vi "GF_Fire_VFandUF.vi"(0 "VF task":refnum<k21>, 1 "Fake Form index":i32, 2 "Preflash Index":i32, 3 "Preflash Width\\Lead":i32=2000, 5 "VF trig array size":i32, 7 "UF task":refnum<k21>, 9 "UF trig array size":i32, 11 "error in":errorcluster, 12 "Spectro Trig Index":i32, 13 "VF Trig Channel":refnum<k21>="USB_TurnOffBProbeRelay_P0_4") -> (15 "error out":errorcluster)   [LabVIEW 2009]
panel:
  out "Very Fast  Fire Waveform":digitalwaveform[](graph)
  out "Ultra Fast  Fire Waveform":digitalwaveform[](graph)
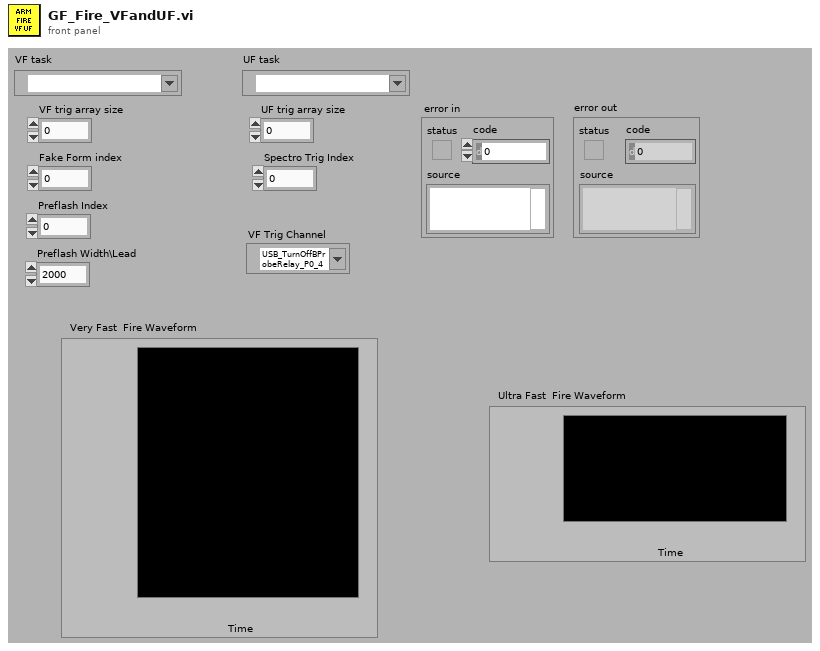
[diagram p1: front panel]
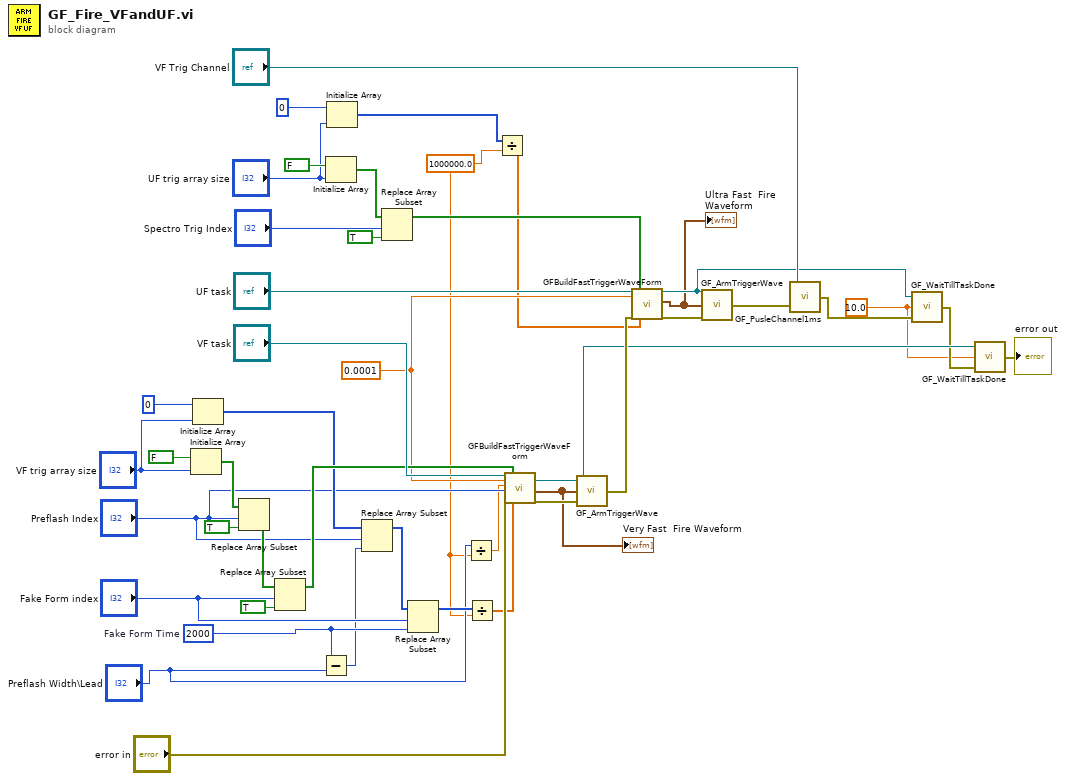
[diagram p0: block diagram]
diagram:
  w2 = 1000000.0 ("Trigger Width")
  w10 = 0.0001 ("Trigger Width")
  w13 = 10.0 ("timeout (sec)")
  w22 = 2000  # Fake Form Time
  n1 = Initialize Array(FALSE, "VF trig array size") -> (w36:bool[])
  n2 = Initialize Array(0, "VF trig array size") -> (w25:i32[])
  n3 = Replace Array Subset(array=w36, new element=TRUE ("new element/subarray"), index="Preflash Index") -> (w35:bool[])
  n4 = Replace Array Subset(array=w35, new element=TRUE ("new element/subarray"), index="Fake Form index") -> (w30:bool[])
  n5 = Subtract(x=w22, y="Preflash Width\\Lead") -> (x-y=w21:i32)
  n6 = Initialize Array(FALSE, "UF trig array size") -> (w38:bool[])
  n7 = Initialize Array(0, "UF trig array size") -> (w7:i32[])
  n8 = Replace Array Subset(array=w25, new element=w21, index="Preflash Index") -> (w24:i32[])
  n9 = Replace Array Subset(array=w38, new element=TRUE ("new element/subarray"), index="Spectro Trig Index") -> (w31:bool[])
  n10 = Replace Array Subset(array=w24, new element=w22, index="Fake Form index") -> (w5:i32[])
  n11 = Divide(x="Preflash Width\\Lead", y=w2) -> (x/y=w1:dbl)
  n12 = Divide(x=w5, y=w2) -> (x/y=w4:dbl[])
  n13 = Divide(x=w7, y=w2) -> (x/y=w6:dbl[])
  n14 = call "GFBuildFastTriggerWaveForm.vi"("task in"="VF task", "Trigger Width"=w10, "Special Trigger Width"=w1, "Special Trig index"="Preflash Index", "error in"="error in", "Enable Array"=w30, "Chan Delays"=w4) -> ("task out"=w15:refnum<k21>, "Digital Waveform Graph"=w9:digitalwaveform[], "error out"=w43:errorcluster)  [unwired: 10 in]
  "Very Fast  Fire Waveform" <- w9
  n15 = call "GF_ArmTriggerWave.vi"("error in"=w43, "trigger waveform"=w9, "task/channels in"=w15) -> ("error out"=w41:errorcluster)
  n16 = call "GFBuildFastTriggerWaveForm.vi"("task in"="UF task", "Trigger Width"=w10, "error in"=w41, "Enable Array"=w31, "Chan Delays"=w6) -> ("task out"=w16:refnum<k21>, "Digital Waveform Graph"=w8:digitalwaveform[], "error out"=w42:errorcluster)  [unwired: 12 in]
  "Ultra Fast  Fire Waveform" <- w8
  n17 = call "GF_ArmTriggerWave.vi"("error in"=w42, "trigger waveform"=w8, "task/channels in"=w16) -> ("error out"=w18:errorcluster)
  n18 = call "GF_PusleChannel1ms.vi"("error in"=w18, "DAQmx Global Channel"="VF Trig Channel") -> ("error out"=w17:errorcluster)
  n19 = call "GF_WaitTillTaskDone.vi"("error in"=w17, "timeout (sec)"=w13, "task/channels in"=w16) -> ("error out"=w14:errorcluster)
  n20 = call "GF_WaitTillTaskDone.vi"("error in"=w14, "timeout (sec)"=w13, "task/channels in"=w15) -> ("error out"=→"error out":errorcluster)
